vi "LED Config (3 colors built in)vi.vi"(8 "refnum name":string, 9 "Channel C":bool, 10 "Channel B":bool, 11 "Channel A":bool) -> ()   [LabVIEW 2019]
uses:
  <vilib>/Rock Robotics/WPI/ThirdParty/Phoenix-LabVIEW/CANifier/CTRE_CANifier_LEDChannel.ctl
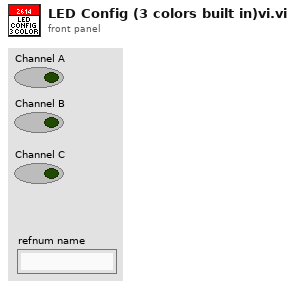
[diagram p1: front panel]
types:
  T1 = typedef "CTRE_CANifier_LEDChannel.ctl" = enum32{"LEDChannelA", "LEDChannelB", "LEDChannelC"}
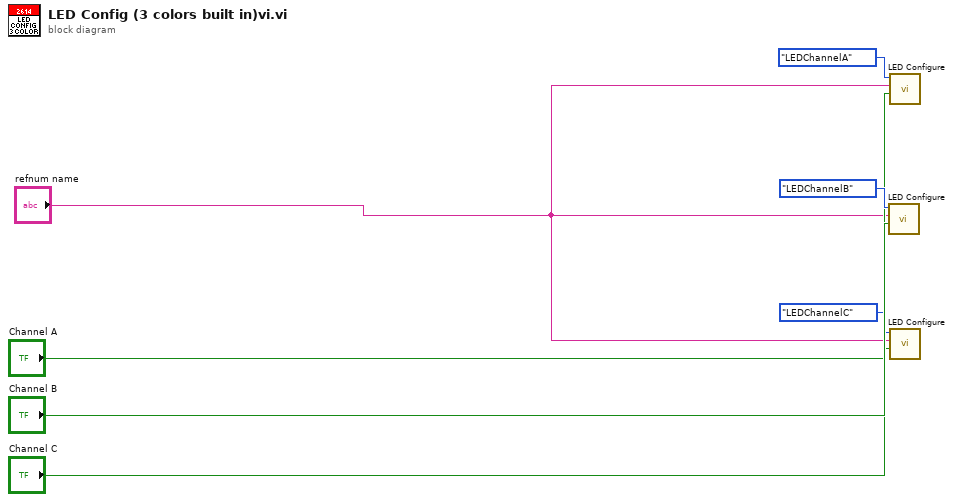
[diagram p0: block diagram]
diagram:
  n1 = call "LED Configure.vi"("LED On"="Channel B", "refnum name"="refnum name", "LEDChannel"=CTRE_CANifier_LEDChannel."LEDChannelB") -> ()  [unwired: 9 in]
  n2 = call "LED Configure.vi"("LED On"="Channel A", "refnum name"="refnum name", "LEDChannel"=CTRE_CANifier_LEDChannel."LEDChannelA") -> ()  [unwired: 9 in]
  n3 = call "LED Configure.vi"("LED On"="Channel C", "refnum name"="refnum name", "LEDChannel"=CTRE_CANifier_LEDChannel."LEDChannelC") -> ()  [unwired: 9 in]
